vi "Switch_sub.vi"(7 "ON":bool, 8 "error in":errorcluster, 9 "PORT":dbl=1.0 min=1.0 max=4.0 step=1.0, 10 "MASTER":dbl=1.0 min=1.0 max=10.0 step=1.0, 11 "IP":string="192.168.23.100") -> (0 "error out":errorcluster)   [LabVIEW 2022 SP3]
uses:
  <vilib>/NI/Advanced HTTP Client/POST (Buffer).vi
  <vilib>/NI/Advanced HTTP Client/Session.lvclass
panel:
  # "Smart connector switch on / off"
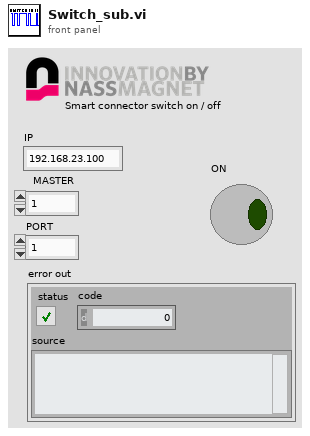
[diagram p1: front panel]
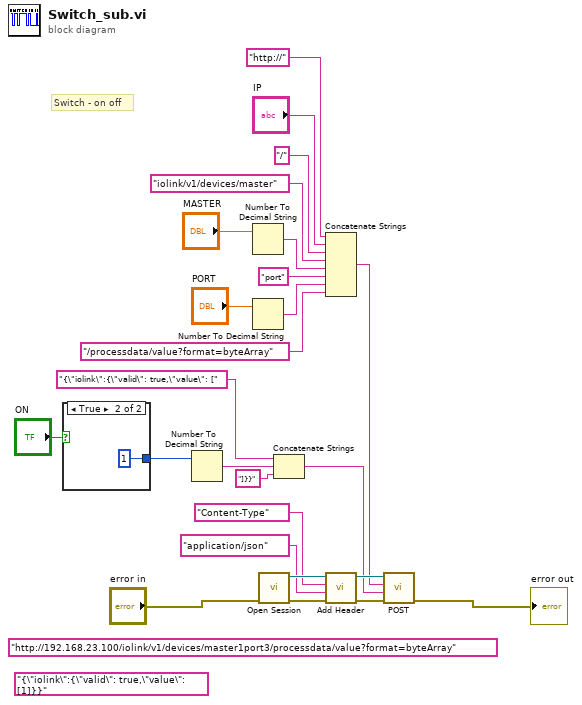
[diagram p0: block diagram]
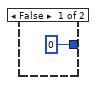
[diagram p2: hidden frame]
diagram:
  (unwired) "{\"iolink\":{\"valid\": true,\"value\": [1]}}" ("buffer")
  (unwired) "http://192.168.23.100/iolink/v1/devices/master1port3/processdata/value?format=byteArray" ("url")
  # "Switch - on off"
  n1 = case shown="True" "ON" {
    tunnel: [0 1] -> w7
    frame False {
    }
    frame True {
    }
  }
  n2 = Number To Decimal String(number=w7) -> (decimal integer string=w6:string)  [unwired: 1 in]
  n3 = Number To Decimal String(number="MASTER") -> (decimal integer string=w13:string)  [unwired: 1 in]
  n4 = Number To Decimal String(number="PORT") -> (decimal integer string=w11:string)  [unwired: 1 in]
  n5 = call <vilib>:"Open Session.vi"("error in"="error in") -> ("error out"=w24:errorcluster, "session"=w25:refnum<class "Session.lvclass">)  [unwired: 9 in]
  n6 = Concatenate Strings("{\"iolink\":{\"valid\": true,\"value\": [" ("string"), w6, "]}}" ("string")) -> (w3:string)
  n7 = Concatenate Strings("http://" ("string"), "IP", "/" ("string"), "iolink/v1/devices/master" ("string"), w13, "port" ("string"), w11, "/processdata/value?format=byteArray" ("string")) -> (w9:string)
  n8 = call <vilib>:"Add Header.vi"("error in"=w24, "value"="application/json" ("buffer"), "header"="Content-Type", "session in"=w25) -> ("error out"=w20:errorcluster, "session out"=w21:refnum<class "Session.lvclass">)  [unwired: 6 in]
  n9 = call-poly <vilib>:"POST.vi"("error in"=w20, "buffer"=w3, "url"=w9, "session in"=w21) -> ("error out"=→"error out":errorcluster)  [unwired: 3 in, 4 out]
